vi "Test Process Log Started Lifecycle State.vi"(8 "error in (no error)":errorcluster, 11 "Process Test In":refnum<class "Process Dev Test.lvclass">) -> (0 "error out":errorcluster, 3 "Process Test Out":refnum<class "Process Dev Test.lvclass">)   [LabVIEW 2020, in "Process Dev Test.lvclass"]
uses:
  Process Dev Test.lvclass
  C:/Program Files (x86)/National Instruments/LabVIEW 2020/vi.lib/Astemes/LUnit/Test Case.lvclass
  source/Framework Test Suite/Mock Log Handler/Mock Log Handler.lvclass
  C:/Git/astemes-triarc-framework/source/Framework/Logging/Logging.lvclass
  source/Framework/Process/Process.lvclass/Process.ctl
  <vilib>/Astemes/LUnit/Test Case.lvclass/Test Case.ctl
  <vilib>/Astemes/LUnit/LUnit Assertion Result.lvclass/LUnit Assertion Result.ctl
  <vilib>/Astemes/LUnit/LUnit Test Case Result.lvclass/LUnit Test Case Result.ctl
  <vilib>/Astemes/LUnit/LUnit Method Result.lvclass/LUnit Method Result.ctl
  63cd48a4-71ab-406d-8512-4a07cc0c0a64.vi
  source/Framework/Process/Public/Lifecycle/Get Lifecycle State.vi
  source/Framework/Process/Protected/Messaging/Send Message.vi
  <vilib>/Astemes/LUnit/Palette/Pass.vi
  <vilib>/Astemes/LUnit/Palette/Fail.vi
  <vilib>/Astemes/LUnit/Compare Variants.vi
  <vilib>/Astemes/LUnit/Describe Comparison.vi
  <vilib>/Astemes/LUnit/Set Assertion Type.vi
  source/Framework/Process/Private/SubVIs/Wait for finish.vi
  source/Framework/Process/Private/SubVIs/Set Lifecycle State.vi
  <vilib>/Utility/error.llb/Clear Errors.vi
  source/Framework/Process/Private/SubVIs/Handle Debug Data.vi
  <vilib>/Astemes/LUnit/Add test result.vi
  <vilib>/Astemes/LUnit/LUnit Write Passed.vi
  <vilib>/Astemes/LUnit/LUnit Write Message.vi
  <vilib>/Astemes/LUnit/LUnit Write Description.vi
  <vilib>/Astemes/LUnit/Variant to string.vi
  <vilib>/Astemes/LUnit/LUnit Write Assertion Type.vi
  source/Framework/Logging/Log Debug.vi
  <vilib>/AdvancedString/1D String Array to Delimited String.vi
  <vilib>/Utility/High Resolution Relative Seconds.vi
  <vilib>/Astemes/LUnit/LUnit Record Assertion Result.vi
  <vilib>/Astemes/LUnit/LUnit Aggregate Assertion Results.vi
  <vilib>/Astemes/LUnit/Assertion Result/LUnit Read Status.vi
  <vilib>/Astemes/LUnit/LUnit Read Message.vi
  <vilib>/Astemes/LUnit/LUnit Read Description.vi
  <vilib>/Astemes/LUnit/Method Result/LUnit Merge Status.vi
  <vilib>/Astemes/LUnit/LUnit Concatenate result strings.vi
  <vilib>/Utility/error.llb/Error Cluster From Error Code.vi
  source/Framework/Process/Public/Read Name.vi
  <vilib>/Utility/Data Type/Get Type Information.vi
  <vilib>/Utility/LVClass/Get LV Class Name.vi
  <vilib>/Astemes/LUnit/LUnit Assertion Result.lvclass
  source/Framework/Process/Process.lvclass
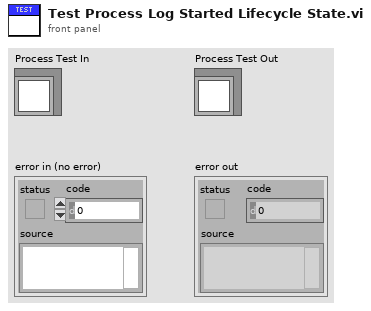
[diagram p1: front panel]
types:
  T1 = typedef "Mock Log Handler.lvclass/Log Entry.ctl" = cluster{"Level":string, "Source":string, "Message":string}
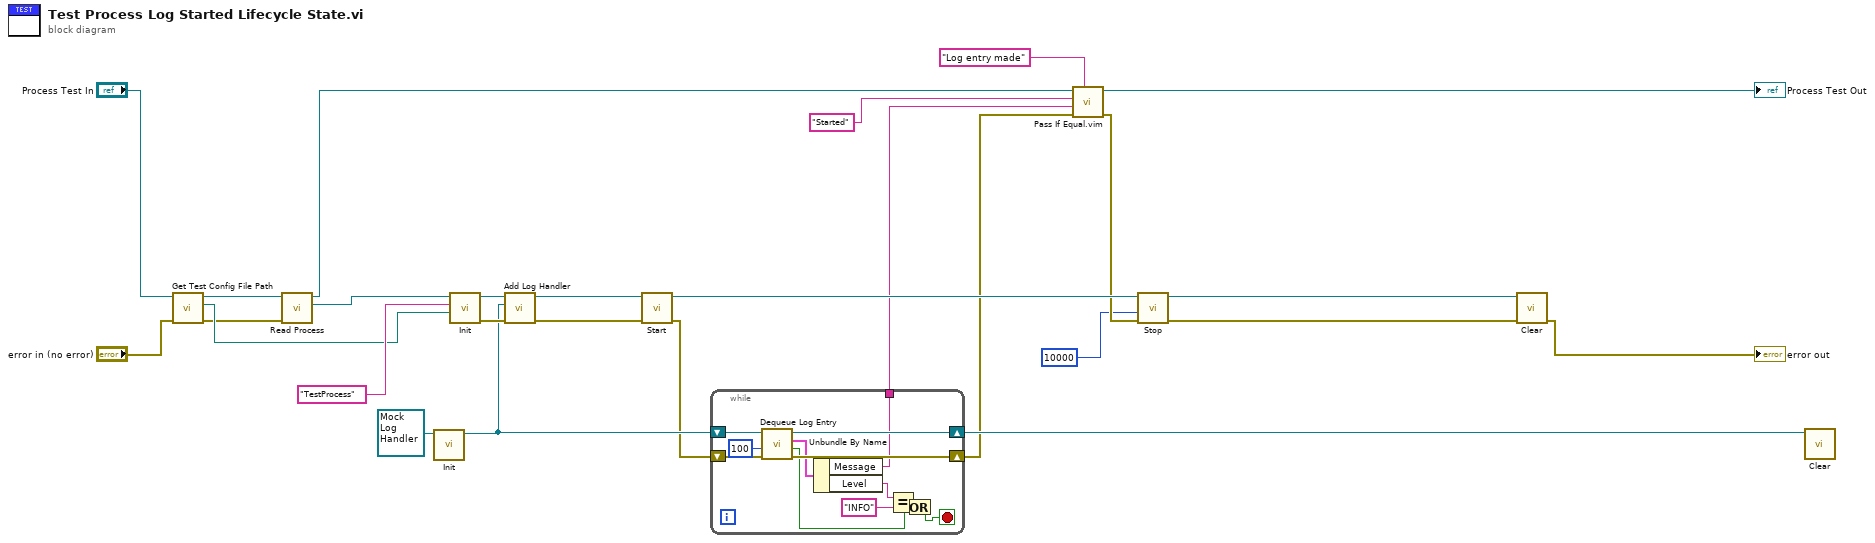
[diagram p0: block diagram]
diagram:
  n1 = call "Get Test Config File Path.vi"("error in (no error)"="error in (no error)", "Process Test In"="Process Test In") -> ("error out"=w12:errorcluster, "Test config path"=w16:path, "Process Test Out"=w14:refnum<class "Process Dev Test.lvclass">)  [unwired: 7 in]
  n2 = call "Read Process.vi"("error in (no error)"=w12, "Process Test in"=w14) -> ("Process.lvclass"=w13:refnum<class "Process.lvclass">, "Process Test out"=w10:refnum<class "Process Dev Test.lvclass">)  [unwired: 7 in, 1 out]
  n3 = call-dynamic "Init.vi"("Mock Log Handler In"=refnum<class "Mock Log Handler.lvclass"> refnum) -> ("Mock Log Handler Out"=w6:refnum<class "Mock Log Handler.lvclass">)  [unwired: 9 in, 1 out]
  n4 = call-dynamic "Init.vi"("Config File Path"=w16, "Name"="TestProcess", "Process In"=w13) -> ("error out"=w27:errorcluster, "Process Out"=w8:refnum<class "Process.lvclass">)  [unwired: 7 in]
  n5 = call "Add Log Handler.vi"("error in (no error)"=w27, "Log Handler"=w6, "Process In"=w8) -> ("error out"=w20:errorcluster, "Process Out"=w26:refnum<class "Process.lvclass">)  [unwired: 7 in]
  n6 = call "Start.vi"("error in (no error)"=w20, "Process In"=w26) -> ("error out"=w4:errorcluster, "Process Out"=w25:refnum<class "Process.lvclass">)  [unwired: 7 in, 1 out]
  n7 = while {
    shift-right: [w38] -> w5
    shift-left: w6 -> [w39]
    shift-right: [w36] -> w3
    shift-left: w4 -> [w37]
    tunnel: [w31] -> w2
    stop <- w29 stop-if-true
    n8 = call "Dequeue Log Entry.vi"("error in (no error)"=w37, "timeout in ms (-1)"=100, "Mock Log Handler in"=w39) -> ("error out"=w36:errorcluster, "timed out?"=w28:bool, "Entry"=w34:T1, "Mock Log Handler out"=w38:refnum<class "Mock Log Handler.lvclass">)  [unwired: 5 in]
    n9 = Unbundle By Name(w34) -> ("Message"=w31:string, "Level"=w33:string)
    n10 = Equal?(x=w33, y="INFO") -> (x = y?=w35:bool)
    n11 = Or(x=w35, y=w28) -> (x .or. y?=w29:bool)
  }
  n12 = call "Pass If Equal.vim"("Description"="Log entry made", "error in (no error)"=w3, "Actual"=w2, "Expected"="Started", "LUnit Test Case In"=w10) -> ("error out"=w19:errorcluster, "LUnit Test Case Out"=→"Process Test Out":refnum<class "Process Dev Test.lvclass">)  [unwired: 5 in]
  n13 = call "Stop.vi"("error in (no error)"=w19, "timeout in ms (-1)"=10000, "Process In"=w25) -> ("error out"=w15:errorcluster, "Process Out"=w24:refnum<class "Process.lvclass">)  [unwired: 6 in, 1 out]
  n14 = call-dynamic "Clear.vi"("error in (no error)"=w15, "Process In"=w24) -> ("error out"=→"error out":errorcluster)  [unwired: 9 in]
  n15 = call-dynamic "Clear.vi"("Mock Log Handler In"=w5) -> ()  [unwired: 10 in, 1 out]
